vi "hpanel_DO_connect_to_hydraharp.vi"(5 "ui_events":T1, 7 "update_hydraharp_status":refnum<user-event>, 8 "error in (no error)":errorcluster, 9 "Mode":T6 items=["T2"=2, "T3"=3], 10 "Hydraharp Settings":T2 {"CH 8"."ch_offs" min=-99999 max=99999 step=1; "CH 8"."ch_ZeroX" min=0 max=20 step=1; "CH 8"."ch_level" min=0 max=800 step=1; "CH 7"."ch_offs" min=-99999 max=99999 step=1; "CH 7"."ch_ZeroX" min=0 max=20 step=1; "CH 7"."ch_level" min=0 max=800 step=1; "CH 6"."ch_offs" min=-99999 max=99999 step=1; "CH 6"."ch_ZeroX" min=0 max=20 step=1; "CH 6"."ch_level" min=0 max=800 step=1; "CH 5"."ch_offs" min=-99999 max=99999 step=1; "CH 5"."ch_ZeroX" min=0 max=20 step=1; "CH 5"."ch_level" min=0 max=800 step=1; "binning" min=0 max=10 step=1; "CH 4"."ch_offs" min=-99999 max=99999 step=1; "CH 4"."ch_ZeroX" min=0 max=20 step=1; "CH 4"."ch_level" min=0 max=800 step=1; "CH 3"."ch_offs" min=-99999 max=99999 step=1; "CH 3"."ch_ZeroX" min=0 max=20 step=1; "CH 3"."ch_level" min=0 max=800 step=1; "CH 2"."ch_offs" min=-99999 max=99999 step=1; "CH 2"."ch_ZeroX" min=0 max=20 step=1; "CH 2"."ch_level" min=0 max=800 step=1; "CH 1"."ch_offs" min=-99999 max=99999 step=1; "CH 1"."ch_ZeroX" min=0 max=20 step=1; "CH 1"."ch_level" min=0 max=800 step=1; "Sync Settings"."snc_offs" min=-99999 max=99999 step=1; "Sync Settings"."snc_ZeroX" min=0 max=20 step=1; "Sync Settings"."snc_level" min=0 max=800 step=10}, 11 "hydraharp_panel in":refnum<class "hydraharp_panel.lvclass">) -> (0 "error out":errorcluster, 3 "hydraharp_panel out":refnum<class "hydraharp_panel.lvclass">)   [LabVIEW 2015, in "hydraharp_panel.lvclass"]
uses:
  hydraharp_panel.lvclass
  hpanel_acq_modes.ctl
  hpanel_hydraharp_settings.ctl
  hpanel_sync_settings.ctl
  hpanel_sync_div.ctl
  hpanel_channel_settings.ctl
  UI/front_panel_class/ui_user_events.ctl
  hydraharp/hydraharp.lvclass
  hydraharp/hydraharp.lvclass/hydraharp.ctl
  UI/panel_class/panel.lvclass
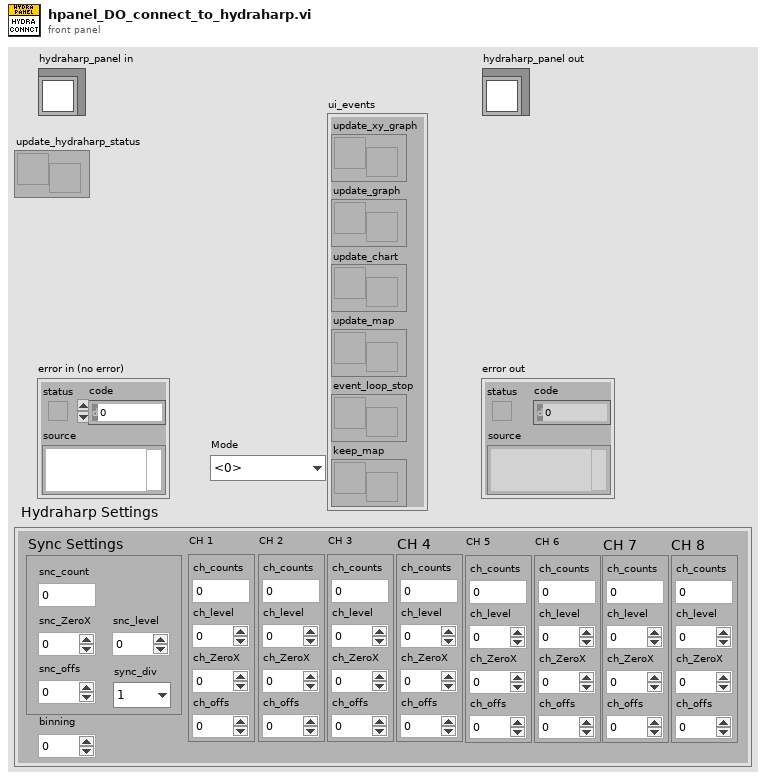
[diagram p1: front panel]
types:
  T1 = typedef "ui_user_events.ctl" = cluster{"update_xy_graph":refnum<user-event>, "update_graph":refnum<user-event>, "update_chart":refnum<user-event>, "update_map":refnum<user-event>, "event_loop_stop":refnum<user-event>, "keep_map":refnum<user-event>}
  T2 = typedef "hpanel_hydraharp_settings.ctl" = cluster{"Sync Settings":T3, "CH 1":T5, "CH 2":T5, "CH 3":T5, "CH 4":T5, "binning":i32, "CH 5":T5, "CH 6":T5, "CH 7":T5, "CH 8":T5}
  T3 = typedef "hpanel_sync_settings.ctl" = cluster{"snc_count":i32, "snc_level":i32, "snc_ZeroX":i32, "snc_offs":i32, "sync_div":T4}
  T4 = typedef "hpanel_sync_div.ctl" = enum16{"1", "2", "4", "8"}
  T5 = typedef "hpanel_channel_settings.ctl" = cluster{"ch_counts":i32, "ch_level":i32, "ch_ZeroX":i32, "ch_offs":i32}
  T6 = typedef "hpanel_acq_modes.ctl" = u16
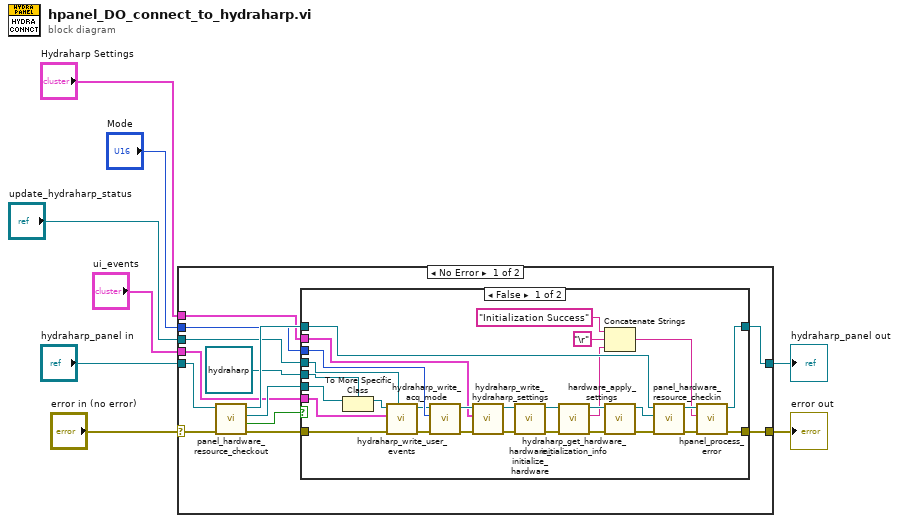
[diagram p0: block diagram]
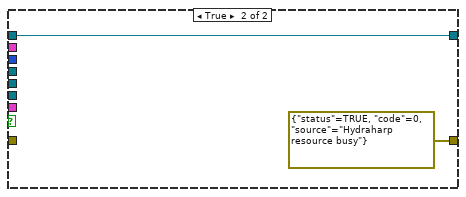
[diagram p2: hidden frame]
diagram:
  n1 = case shown="No Error" "error in (no error)" {
    selector: "error in (no error)" -> [w20 w54]
    tunnel: [w17 w54] -> w7
    tunnel: [w11 w53] -> w5
    tunnel: "hydraharp_panel in" -> [w21 w53]
    tunnel: "Mode" -> [w13 _]
    tunnel: "Hydraharp Settings" -> [w12 _]
    tunnel: "update_hydraharp_status" -> [w10 _]
    tunnel: "ui_events" -> [w9 _]
    frame No Error {
      n2 = call "panel_hardware_resource_checkout.vi"("error in (no error)"=w20, "panel in"=w21) -> ("error out"=w18:errorcluster, "timed out?"=w19:bool, "hardware.lvclass"=w15:refnum<class "hardware.lvclass">, "panel out"=w16:refnum<class "hydraharp_panel.lvclass">)  [unwired: 6 in]
      n3 = case shown="False" w19 {
        tunnel: w18 -> [w35 _]
        tunnel: [w23 errorcluster {"status"=TRUE, "code"=0, "source"="Hydraharp resource busy"} ("error out")] -> w17
        tunnel: w16 -> [w42 w51]
        tunnel: w15 -> [w49 _]
        tunnel: refnum<class "hydraharp.lvclass"> refnum ("hydraharp.lvclass") -> [w50 _]
        tunnel: w13 -> [w44 _]
        tunnel: w12 -> [w43 _]
        tunnel: [w22 w51] -> w11
        tunnel: w10 -> [w31 _]
        tunnel: w9 -> [w30 _]
        frame False {
          n4 = To More Specific Class(target class=w50, reference=w49) -> (specific class reference=w33:refnum<class "hydraharp.lvclass">)  [unwired: 1 in, 1 out]
          n5 = call "hydraharp_write_user_events.vi"("update_hydraharp_status"=w31, "error in (no error)"=w35, "ui_events"=w30, "hydraharp in"=w33) -> ("error out"=w34:errorcluster, "hydraharp out"=w32:refnum<class "hydraharp.lvclass">)  [unwired: 6 in]
          n6 = call "hydraharp_write_acq_mode.vi"("error in (no error)"=w34, "Mode"=w44, "hydraharp in"=w32) -> ("error out"=w47:errorcluster, "hydraharp out"=w48:refnum<class "hydraharp.lvclass">)  [unwired: 7 in]
          n7 = call "hydraharp_write_hydraharp_settings.vi"("error in (no error)"=w47, "Hydraharp Settings"=w43, "hydraharp in"=w48) -> ("error out"=w46:errorcluster, "hydraharp out"=w45:refnum<class "hydraharp.lvclass">)  [unwired: 7 in]
          n8 = call-dynamic "hardware_initialize_hardware.vi"("error in (no error)"=w46, "hydraharp in"=w45) -> ("error out"=w40:errorcluster, "hydraharp out"=w41:refnum<class "hydraharp.lvclass">)  [unwired: 8 in]
          n9 = call "hydraharp_get_hardware_initialization_info.vi"("error in (no error)"=w40, "hydraharp in"=w41) -> ("error out"=w38:errorcluster, "resulting string"=w27:string, "hydraharp out"=w39:refnum<class "hydraharp.lvclass">)  [unwired: 7 in]
          n10 = Concatenate Strings("Initialization Success" ("String"), "\r", w27) -> (w24:string)
          n11 = call-dynamic "hardware_apply_settings.vi"("error in (no error)"=w38, "hydraharp in"=w39) -> ("error out"=w37:errorcluster, "hydraharp out"=w36:refnum<class "hydraharp.lvclass">)  [unwired: 8 in]
          n12 = call "panel_hardware_resource_checkin.vi"("error in (no error)"=w37, "hardware.lvclass"=w36, "panel in"=w42) -> ("error out"=w26:errorcluster, "panel out"=w25:refnum<class "hydraharp_panel.lvclass">)  [unwired: 7 in]
          n13 = call "hpanel_process_error.vi"("error in (no error)"=w26, "No Error Message"=w24, "hydraharp_panel in"=w25) -> ("error out"=w23:errorcluster, "hydraharp_panel out"=w22:refnum<class "hydraharp_panel.lvclass">)  [unwired: 7 in]
        }
        frame True {
        }
      }
    }
    frame Error {
    }
  }
  "error out" <- w7
  "hydraharp_panel out" <- w5
